vi "LoadDataKen.vi"(5 "Path":refnum<vi>) -> ()   [LabVIEW 2009]
panel:
  out "% done":dbl(slide) scale=0.0..100.0
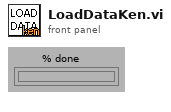
[diagram p1: front panel]
types:
  T1 = cluster{"router channels":u8[], "macro times":dbl[], "micro times":u16[], "invalid times":dbl[], "gap times":dbl[]}
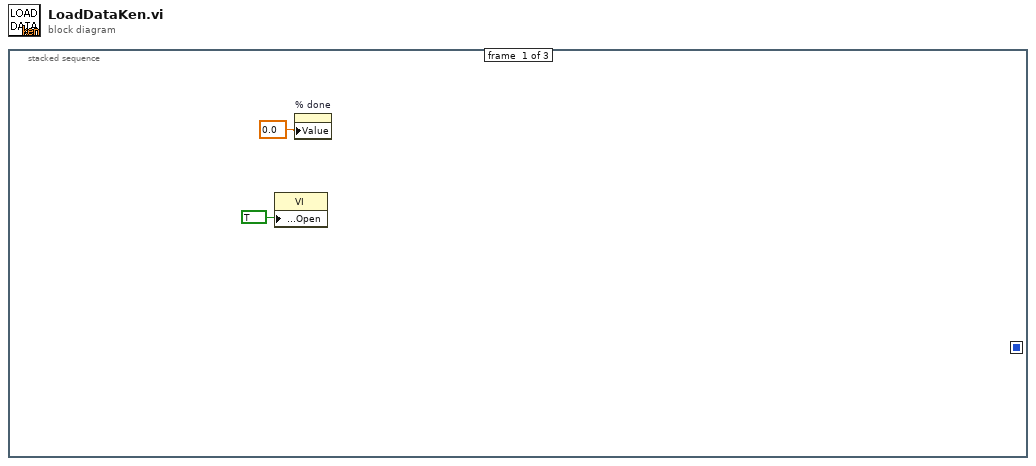
[diagram p0: block diagram]
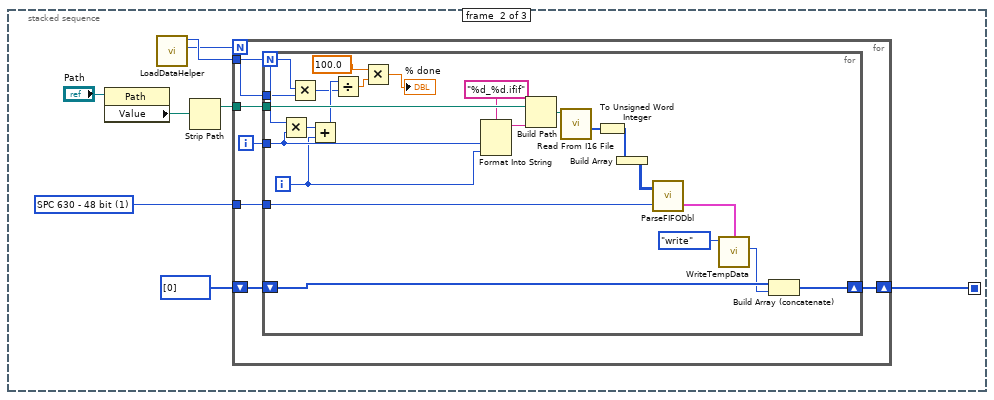
[diagram p2: hidden frame]
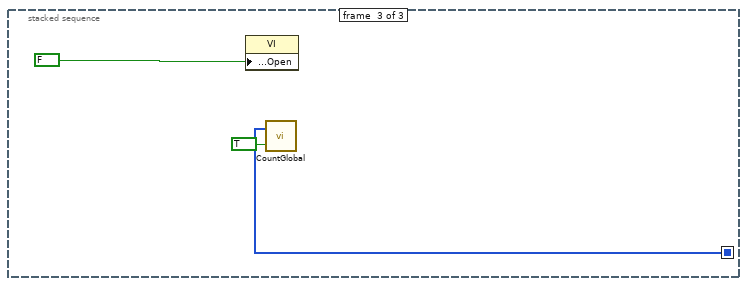
[diagram p3: hidden frame]
diagram:
  n1 = stacked-sequence {
    seq-local: [_ w7 _] -> [_ _ w43]
    frame #0 {
      n2 = property class="VI"("Front Panel Window:Open"=TRUE) -> ()  [unwired: 2 in, 2 out]
      n3 = property on="% done" class="Slide (strict)"("Value"=0.0 ("% done")) -> ()  [unwired: 2 in, 2 out]
    }
    frame #1 {
      w3 = u16 1 items=["SPC 630 - 32 bit", "SPC 630 - 48 bit", "SPC 830 - 32 bit", "SPC 130 - 32 bit", ""] ("SPC Format")
      n4 = property on="Property Node" class="Path"(reference="Path") -> ("Value"=w10:path)  [unwired: 1 in, 2 out]
      n5 = call "LoadDataHelper.vi"() -> ("planes"=w5:u32, "lines"=w6:u32)  [unwired: 7 in, 3 out]
      n6 = Strip Path(path=w10) -> (stripped path=w9:path)  [unwired: 1 out]
      n7 = for {
        N: w5 -> [w11]
        tunnel: w6 -> [w14]
        tunnel: w9 -> [w17]
        tunnel: w3 -> [w15]
        shift-right: [w12] -> w7
        shift-left: i32[] [0] -> [w13]
        i -> [w16]
        n8 = for {
          N: w14 -> [w29]
          tunnel: w17 -> [w40]
          tunnel: w16 -> [w30]
          tunnel: w15 -> [w22]
          shift-right: [w38] -> w12
          shift-left: w13 -> [w39]
          tunnel: w11 -> [w25]
          i -> [w28]
          n9 = Multiply(x=w29, y=w30) -> (x*y=w26:i32)
          n10 = Multiply(x=w29, y=w25) -> (x*y=w24:i32)
          n11 = Add(x=w26, y=w28) -> (x+y=w27:i32)
          n12 = Divide(x=w27, y=w24) -> (x/y=w31:dbl)
          n13 = Multiply(x=100.0, y=w31) -> (x*y=→"% done":dbl)
          n14 = Format Into String(format string="%d_%d.ifif", w30, w28) -> (resulting string=w34:string)  [unwired: 2 in, 1 out]
          n15 = Build Path(base path=w40, name or relative path=w34) -> (appended path=w33:path)
          n16 = call "Read From I16 File.vi"("file path (dialog if empty)"=w33) -> ("1D array"=w32:i16[])  [unwired: 6 in, 4 out]
          n17 = To Unsigned Word Integer(number=w32) -> (unsigned 16bit integer=w23:u16[])
          n18 = Build Array(w23) -> (w21:u16[][])
          n19 = call "ParseFIFODbl.vi"("SPC Format"=w22, "FIFO rawdata"=w21) -> ("rawdata"=w19:T1)  [unwired: 1 in]
          n20 = call "WriteTempData.vi"("rawdata"=w19, "Enum"=enum16{"create new", "write", "close"}."write") -> ("offset"=w18:i32)  [unwired: 3 in, 1 out]
          n21 = Build Array (concatenate)(w39, w18) -> (w38:i32[])
        }
      }
    }
    frame #2 {
      n22 = property class="VI"("Front Panel Window:Open"=FALSE) -> ()  [unwired: 2 in, 2 out]
      n23 = call "CountGlobal.vi"("changed?"=TRUE, "count"=w43) -> ()  [unwired: 1 in, 1 out]
    }
  }
